vi "ScopeTraceFGV.vi"(9 "output waveform":waveform(dbl), 10 "command":T1, 11 "Nr.":i32) -> (2 "All Channels":waveform(dbl)[](array[waveform]), 3 "Channel":waveform(dbl))   [LabVIEW 2013]
uses:
  commandForScopeTrace.ctl
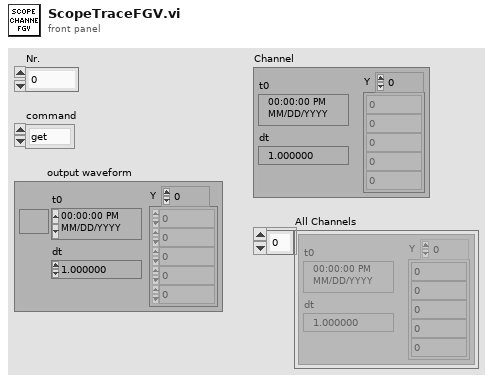
[diagram p1: front panel]
types:
  T1 = typedef "commandForScopeTrace.ctl" = enum16{"get", "set", "init", "get ALL"}
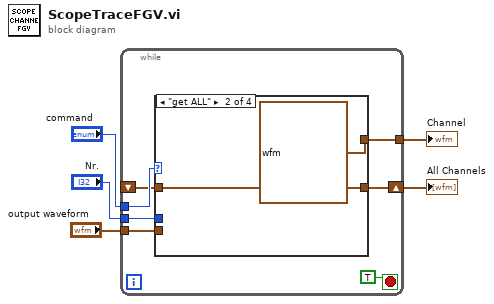
[diagram p0: block diagram]
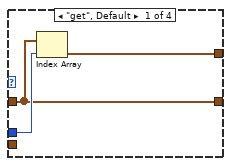
[diagram p2: hidden frame]
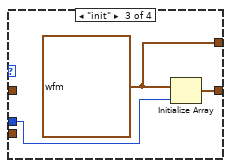
[diagram p3: hidden frame]
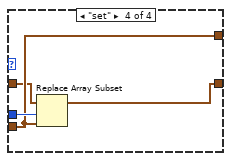
[diagram p4: hidden frame]
diagram:
  n1 = while {
    shift-right: [w9] -> w4
    shift-left: _ -> [w7]
    tunnel: "Nr." -> [w11]
    tunnel: "output waveform" -> [w10]
    tunnel: "command" -> [w8]
    tunnel: [w6] -> w5
    stop <- TRUE stop-if-true
    n2 = case shown="\"get ALL\"" w8 {
      tunnel: w11 -> [w14 _ w18 w24]
      tunnel: w10 -> [_ _ _ w22]
      tunnel: [w13 w17 w20 w23] -> w9
      tunnel: w7 -> [w13 w17 _ w21]
      tunnel: [w15 waveform(dbl) {"t0"=timestamp(0 s since 1904-01-01), "dt"=1.0, "Y"=[]} ("output waveform") w19 w22] -> w6
      frame "get", Default {
        n3 = Index Array(array=w13, index=w14) -> (element=w15:waveform(dbl))
      }
      frame "get ALL" {
      }
      frame "init" {
        w19 = waveform(dbl) {"t0"=timestamp(0 s since 1904-01-01), "dt"=1.0, "Y"=[]} ("output waveform")
        n4 = Initialize Array(w19, w18) -> (w20:waveform(dbl)[])
      }
      frame "set" {
        n5 = Replace Array Subset(array=w21, new element=w22, index=w24) -> (w23:waveform(dbl)[])
      }
    }
  }
  "All Channels" <- w4
  "Channel" <- w5
